vi "Write MotorPWM.vi"(8 "error in (no error)":errorcluster, 10 "MotorPWM":dbl, 11 "Car.lvclass":refnum<class "Car.lvclass">) -> (0 "error out":errorcluster, 3 "Car.lvclass 2":refnum<class "Car.lvclass">)   [LabVIEW 2015, in "Car.lvclass"]
uses:
  Car.lvclass
  Car.lvclass/Car.ctl
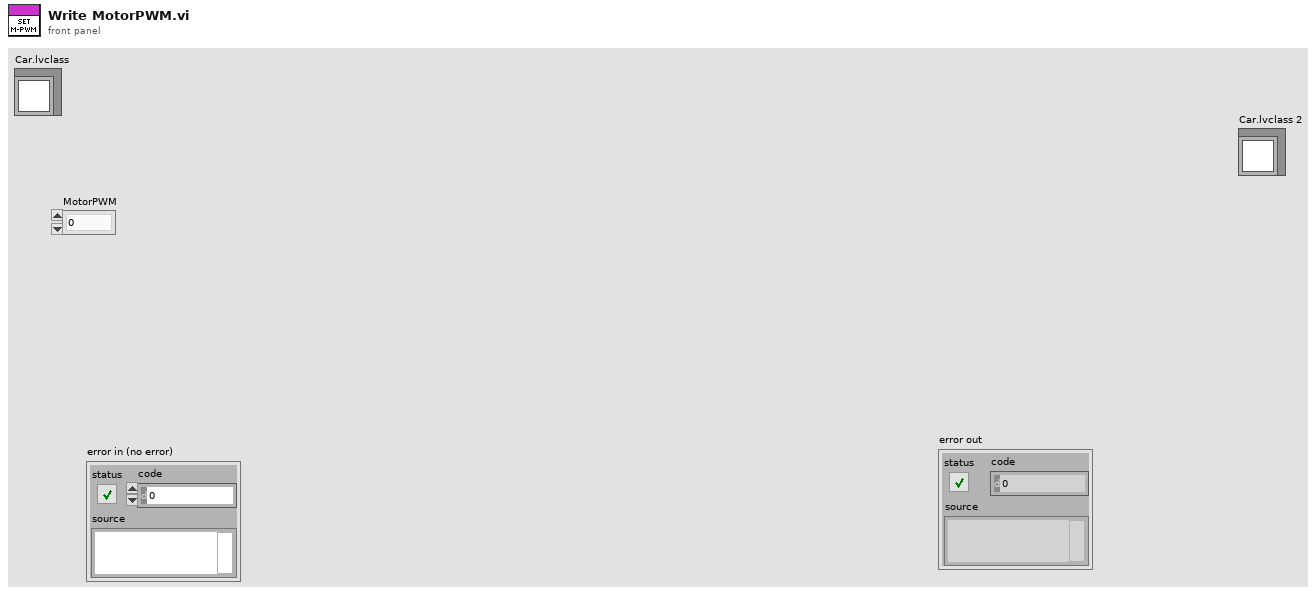
[diagram p1: front panel]
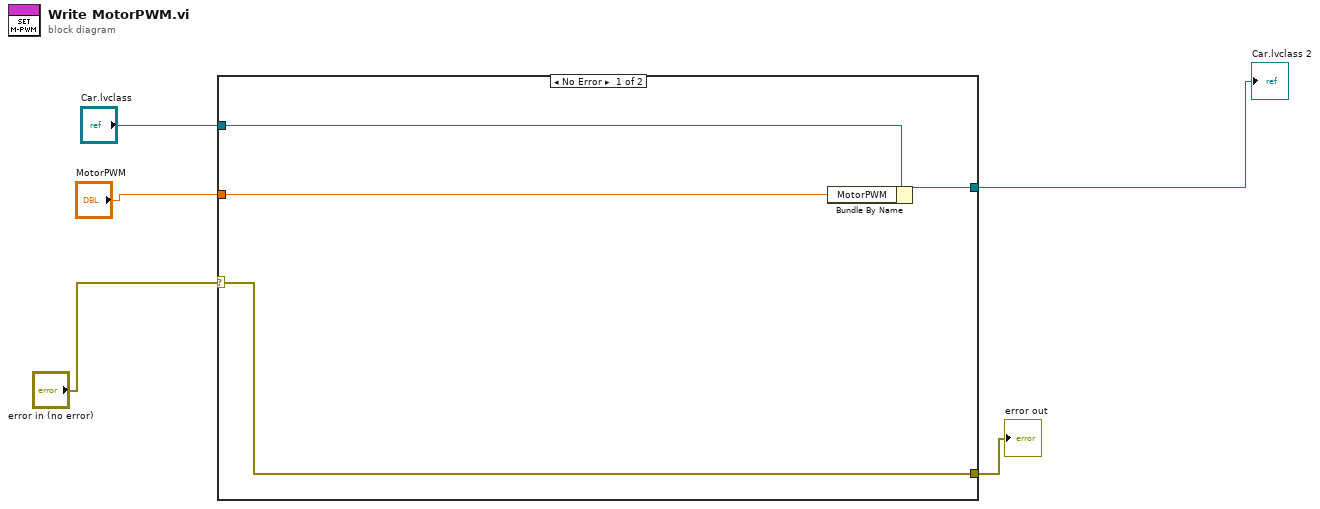
[diagram p0: block diagram]
diagram:
  n1 = case shown="No Error" "error in (no error)" {
    selector: "error in (no error)" -> [w9 w10]
    tunnel: [w9 w10] -> w4
    tunnel: [w7 w11] -> w3
    tunnel: "Car.lvclass" -> [w8 w11]
    tunnel: "MotorPWM" -> [w6 _]
    frame No Error {
      n2 = Bundle By Name(cluster=w8, "MotorPWM"=w6) -> (w7:refnum<class "Car.lvclass">)
    }
    frame Error {
    }
  }
  "Car.lvclass 2" <- w3
  "error out" <- w4
